vi "Insert Side Gyro Data.vi"(4 "Side Gyro Data in":T2, 5 "Data from Gyro":T1) -> (2 "Side Gyro Data out":T2)   [LabVIEW 2019]
uses:
  Controls/Gyro Side Data.ctl
  Controls/Gyro Negation.ctl
  Controls/Data From Gyro.ctl
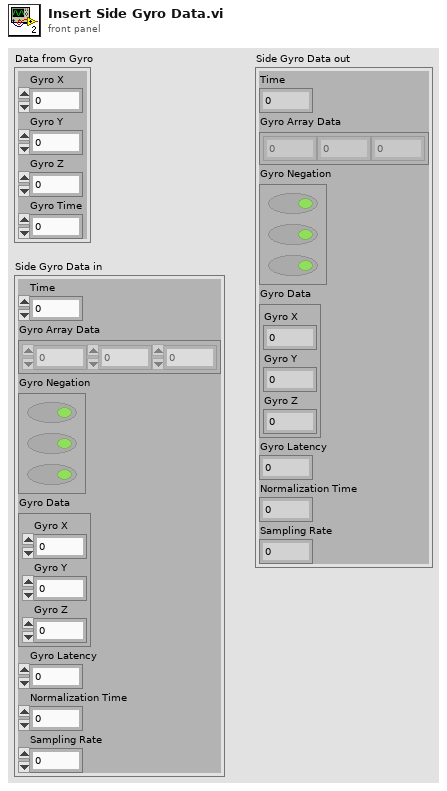
[diagram p1: front panel]
types:
  T1 = typedef "Data From Gyro.ctl" = cluster{"Gyro X":dbl, "Gyro Y":dbl, "Gyro Z":dbl, "Gyro Time":dbl}
  T2 = typedef "Gyro Side Data.ctl" = cluster{"Time":dbl, "Gyro Array Data":dbl[], "Gyro Negation":T3, "Gyro Data":cluster{"Gyro X":dbl, "Gyro Y":dbl, "Gyro Z":dbl}, "Gyro Latency":dbl, "Normalization Time":dbl, "Sampling Rate":dbl}
  T3 = typedef "Gyro Negation.ctl" = bool[]
  T4 = cluster{"Numeric":dbl, "Numeric":dbl, "Numeric":dbl}
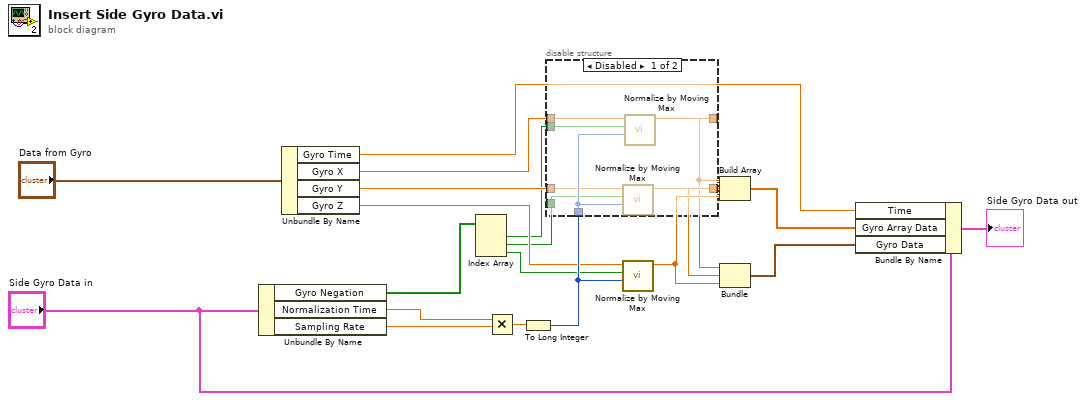
[diagram p0: block diagram]
diagram:
  n1 = Unbundle By Name("Side Gyro Data in") -> ("Gyro Negation"=w1:T3, "Normalization Time"=w3:dbl, "Sampling Rate"=w4:dbl)
  n2 = Unbundle By Name("Data from Gyro") -> ("Gyro Time"=w18:dbl, "Gyro X"=w5:dbl, "Gyro Y"=w8:dbl, "Gyro Z"=w11:dbl)
  n3 = Index Array(array=w1) -> (element #1=w6:bool, element #2=w9:bool, element #3=w12:bool)  [unwired: 3 in]
  n4 = Multiply(x=w3, y=w4) -> (x*y=w2:dbl)
  n5 = To Long Integer(number=w2) -> (32bit integer=w13:i32)
  n6 = disable-structure shown="Disabled" {
    disable-tunnel: w13 -> [w27 _]
    disable-tunnel: [w26 _] -> w10
    disable-tunnel: w9 -> [w25 _]
    disable-tunnel: w8 -> [w24 _]
    disable-tunnel: [w23 _] -> w7
    disable-tunnel: w6 -> [w22 _]
    disable-tunnel: w5 -> [w21 _]
    frame Disabled {
      n7 = call "Normalize by Moving Max.vi"("sample length"=w27, "Negation"=w25, "Value"=w24) -> ("Numeric"=w26:dbl)  [unwired: 4 in]
      n8 = call "Normalize by Moving Max.vi"("sample length"=w27, "Negation"=w22, "Value"=w21) -> ("Numeric"=w23:dbl)  [unwired: 4 in]
    }
    frame Enabled {
    }
  }
  n9 = call "Normalize by Moving Max.vi"("sample length"=w13, "Negation"=w12, "Value"=w11) -> ("Numeric"=w14:dbl)  [unwired: 4 in]
  n10 = Build Array(w7, w10, w14) -> (w16:dbl[])
  n11 = Bundle("Numeric"=w7, "Numeric"=w10, "Numeric"=w14) -> (w17:T4)  [unwired: 1 in]
  n12 = Bundle By Name(cluster="Side Gyro Data in", "Time"=w18, "Gyro Array Data"=w16, "Gyro Data"=w17) -> (→"Side Gyro Data out":T2)
